vi "基于数组的分数查询系统.vi"() -> ()   [LabVIEW 2018]
panel:
  out "数组 2":T1(array[cluster])
  in  "数组":T2(array[cluster])
  out "簇":T3
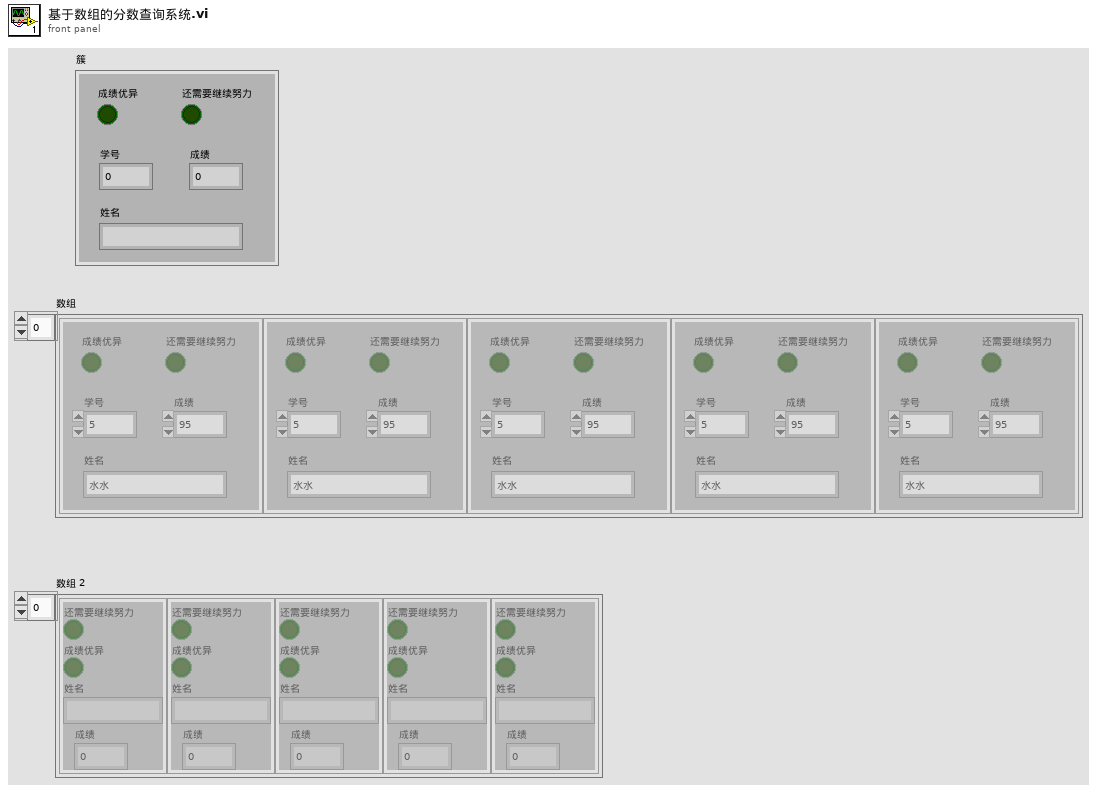
[diagram p1: front panel]
types:
  T1 = cluster{"还需要继续努力":bool, "成绩优异":bool, "姓名":string, "成绩":dbl}[]
  T2 = cluster{"成绩优异":bool, "还需要继续努力":bool, "学号":dbl, "成绩":dbl, "姓名":string}[]
  T3 = cluster{"成绩优异":bool, "还需要继续努力":bool, "学号":dbl, "成绩":dbl, "姓名":string}
  T4 = cluster{"还需要继续努力":bool, "成绩优异":bool, "姓名":string, "成绩":dbl}
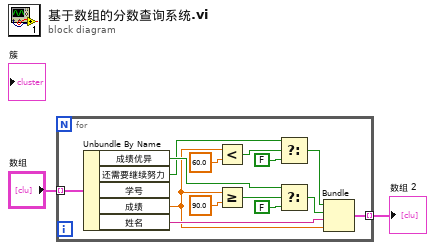
[diagram p0: block diagram]
diagram:
  n1 = for {
    tunnel: "数组" -> [w16] mode=indexing
    tunnel: [w3] -> w1 mode=indexing
    n2 = Unbundle By Name(w16) -> ("成绩优异"=w12:bool, "还需要继续努力"=w5:bool, "成绩"=w9:dbl, "姓名"=w15:string)  [unwired: 1 out]
    n3 = Less?(x=w9, y=60.0 ("x")) -> (x < y?=w6:bool)
    n4 = Greater Or Equal?(x=w9, y=90.0) -> (x >= y?=w13:bool)
    n5 = Select(t=w5, s=w6, f=FALSE) -> (s? t:f=w7:bool)
    n6 = Select(t=w12, s=w13, f=FALSE) -> (s? t:f=w10:bool)
    n7 = Bundle("还需要继续努力"=w7, "成绩优异"=w10, "姓名"=w15, "成绩"=w9) -> (w3:T4)  [unwired: 1 in]
  }
  "数组 2" <- w1
